vi "UserConsole_Queue Driver.vi"(8 "error in (no error)":errorcluster, 10 "State":T1=enum."Init", 11 "EnQ":string) -> (0 "error out":errorcluster, 3 "DeQ":string)   [LabVIEW 2013, in "UserConsole.lvlib"]
uses:
  PrivateControls/UserConsole_QueueDriver.ctl
  UserConsole.lvlib
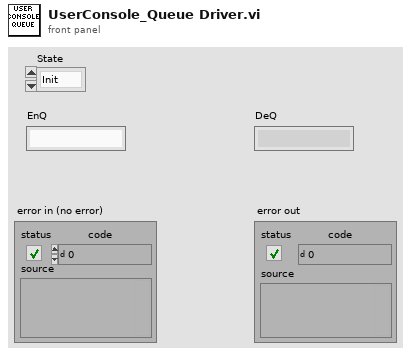
[diagram p1: front panel]
types:
  T1 = typedef "UserConsole.lvlib/UserConsole_QueueDriver.ctl" = enum16{"Default Case", "Init", "Enqueue", "Dequeue", "ReleaseQueue", "Exit"}
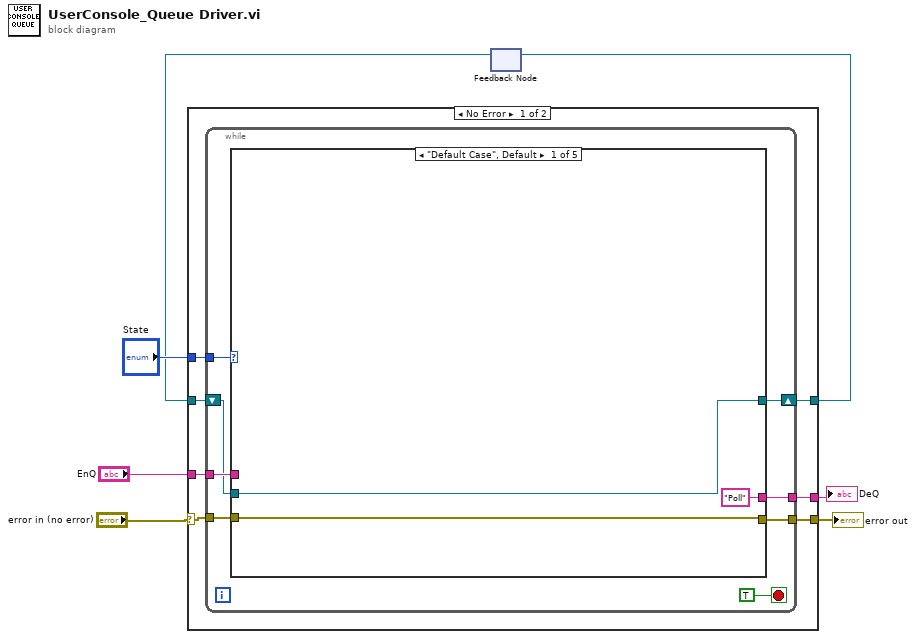
[diagram p0: block diagram]
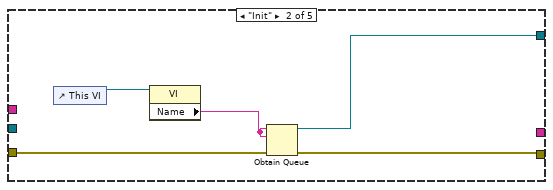
[diagram p2: hidden frame]
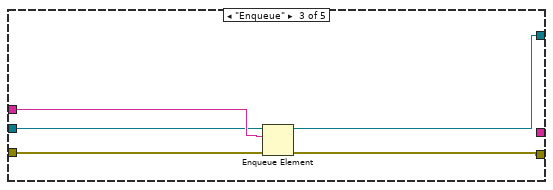
[diagram p3: hidden frame]
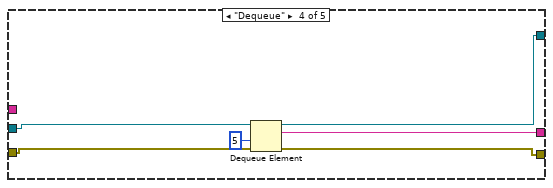
[diagram p4: hidden frame]
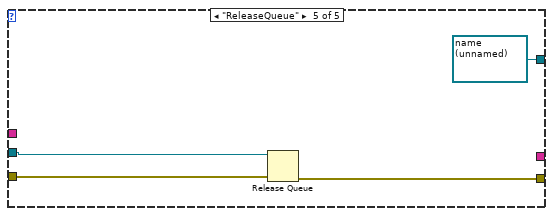
[diagram p5: hidden frame]
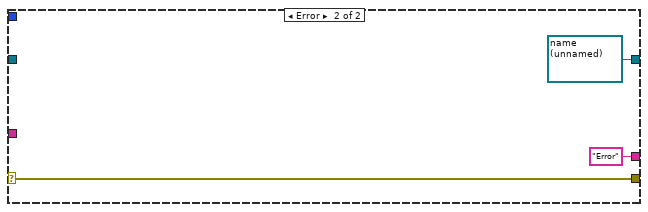
[diagram p6: hidden frame]
diagram:
  n1 = feedback #1() -> (w1:refnum<queue>)  [unwired: 1 in]
  n2 = case shown="No Error" "error in (no error)" {
    selector: "error in (no error)" -> [w12 w48]
    tunnel: [w14 w48] -> w6
    tunnel: "State" -> [w13 _]
    tunnel: "EnQ" -> [w11 _]
    tunnel: [w10 "Error" ("name (unnamed)")] -> w3
    tunnel: [w9 refnum<queue> refnum ("queue out")] -> w2
    tunnel: w1 -> [w8 _]
    frame No Error {
      n3 = while {
        tunnel: [w22] -> w14
        tunnel: w13 -> [w21]
        shift-right: [w20] -> w9
        shift-left: w8 -> [w17]
        tunnel: w12 -> [w19]
        tunnel: w11 -> [w18]
        tunnel: [w16] -> w10
        stop <- TRUE stop-if-true
        n4 = case shown="\"Default Case\", Default" w21 {
          tunnel: [w23 w30 w35 w38 w43] -> w22
          tunnel: [w24 w29 w31 w41 refnum<queue> refnum ("queue out")] -> w20
          tunnel: w19 -> [w23 w28 w34 w37 w44]
          tunnel: w18 -> [_ _ w33 _ _]
          tunnel: w17 -> [w24 _ w32 w40 w45]
          tunnel: ["Poll" ("name (unnamed)") _ _ w39 _] -> w16
          frame "Default Case", Default {
          }
          frame "Init" {
            n5 = control-ref of="This VI"() -> (w27:refnum<vi>)
            n6 = property class="VI"(reference=w27) -> ("Name"=w26:string)  [unwired: 1 in, 2 out]
            n7 = Obtain Queue(name (unnamed)=w26, element data type=w26, error in (no error)=w28) -> (queue out=w29:refnum<queue>, error out=w30:errorcluster)  [unwired: 2 in, 1 out]
          }
          frame "Enqueue" {
            n8 = Enqueue Element(queue=w32, element=w33, error in (no error)=w34) -> (queue out=w31:refnum<queue>, error out=w35:errorcluster)  [unwired: 1 in, 1 out]
          }
          frame "Dequeue" {
            n9 = Dequeue Element(queue=w40, timeout in ms (-1)=5, error in (no error)=w37) -> (queue out=w41:refnum<queue>, element=w39:string, error out=w38:errorcluster)  [unwired: 1 out]
          }
          frame "ReleaseQueue" {
            n10 = Release Queue(queue=w45, error in (no error)=w44) -> (error out=w43:errorcluster)  [unwired: 1 in, 2 out]
          }
        }
      }
    }
    frame Error {
    }
  }
  "error out" <- w6
  "DeQ" <- w3
  n11 = feedback-in #1(w2) -> ()
